vi "fgv_PerfMonBOOL.vi"(7 "FGV Actions":T1, 8 "error in (no error)":errorcluster, 11 "Perf Mon [IN]":bool) -> (0 "error out":errorcluster, 3 "Perf Mon [OUT]":bool)   [LabVIEW 2020]
uses:
  Typedefs/fgv_actions.ctl
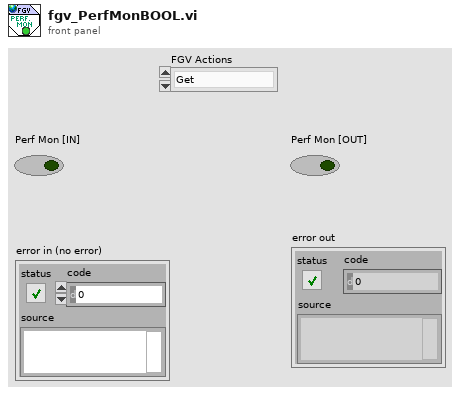
[diagram p1: front panel]
types:
  T1 = typedef "fgv_actions.ctl" = enum16{"Get", "Set"}
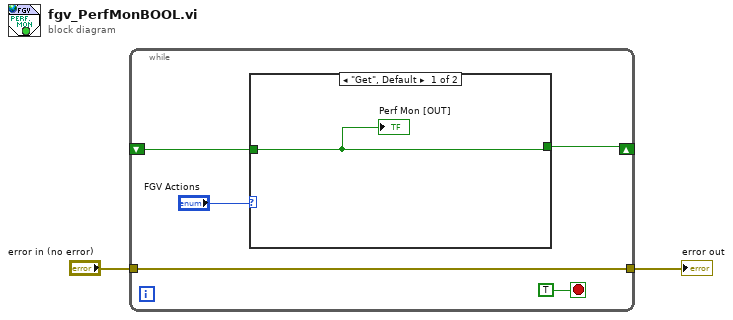
[diagram p0: block diagram]
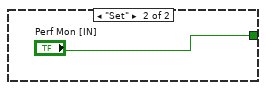
[diagram p2: hidden frame]
diagram:
  n1 = while {
    shift-right: [w5] -> _
    shift-left: _ -> [w4]
    tunnel: "error in (no error)" -> [w3]
    tunnel: [w3] -> w1
    stop <- TRUE stop-if-true
    n2 = case shown="\"Get\", Default" "FGV Actions" {
      tunnel: [w8 "Perf Mon [IN]"] -> w5
      tunnel: w4 -> [w8 _]
      frame "Get", Default {
        "Perf Mon [OUT]" <- w8
      }
      frame "Set" {
      }
    }
  }
  "error out" <- w1
